vi "Is Empty.vi"(8 "error in (no error)":errorcluster, 11 "Interlock Chain in":refnum<class "Interlock Chain.lvclass">) -> (0 "error out":errorcluster, 1 "Is Empty?":bool, 3 "Interlock Chain out":refnum<class "Interlock Chain.lvclass">)   [LabVIEW 2015, in "Interlocks.lvlib" / "Interlock Chain.lvclass"]
uses:
  Interlock Chain.lvclass
  Interlock Chain.lvclass/Interlock Chain.ctl
  Interlock/Interlock.lvclass
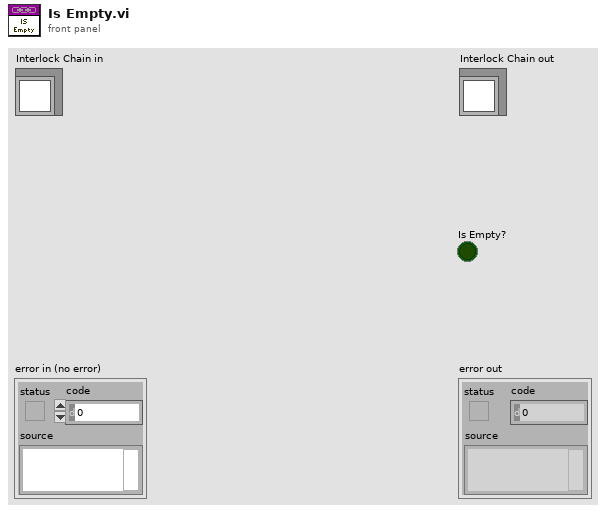
[diagram p1: front panel]
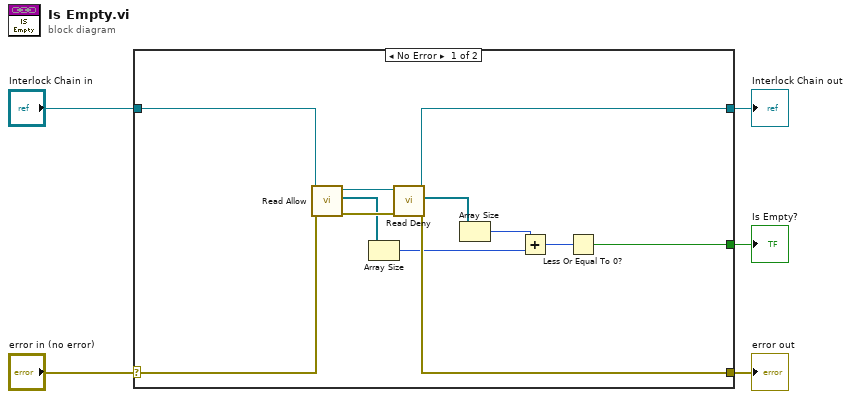
[diagram p0: block diagram]
diagram:
  n1 = case shown="No Error" "error in (no error)" {
    selector: "error in (no error)" -> [w15 w19]
    tunnel: [w14 w19] -> w4
    tunnel: [w12 w18] -> w2
    tunnel: "Interlock Chain in" -> [w13 w18]
    tunnel: [w6 _] -> w1
    frame No Error {
      n2 = call "Read Allow.vi"("error in (no error)"=w15, "Interlock Chain in"=w13) -> ("error out"=w16:errorcluster, "Allow"=w11:refnum<class "Interlock.lvclass">[], "Interlock Chain out"=w17:refnum<class "Interlock Chain.lvclass">)  [unwired: 6 in, 1 out]
      n3 = Array Size(array=w11) -> (size(s)=w9:i32)
      n4 = call "Read Deny.vi"("error in (no error)"=w16, "Interlock Chain in"=w17) -> ("error out"=w14:errorcluster, "Deny"=w10:refnum<class "Interlock.lvclass">[], "Interlock Chain out"=w12:refnum<class "Interlock Chain.lvclass">)  [unwired: 7 in]
      n5 = Array Size(array=w10) -> (size(s)=w8:i32)
      n6 = Add(x=w8, y=w9) -> (x+y=w7:i32)
      n7 = Less Or Equal To 0?(x=w7) -> (x <= 0?=w6:bool)
    }
    frame Error {
    }
  }
  "error out" <- w4
  "Interlock Chain out" <- w2
  "Is Empty?" <- w1
